vi "Read Interrupt.vi"(8 "error in (no error)":errorcluster, 11 "IO-4 Bricklet in":refnum<class "IO-4 Bricklet.lvclass">) -> (0 "error out":errorcluster, 2 "Interrupt":refnum<user-event>, 3 "IO-4 Bricklet out":refnum<class "IO-4 Bricklet.lvclass">)   [LabVIEW 2011, in "Tinkerforge.lvlib" / "IO-4 Bricklet.lvclass"]
uses:
  IO-4 Bricklet.lvclass
  Type Definitions/Interrupt.ctl
  IO-4 Bricklet.lvclass/IO-4 Bricklet.ctl
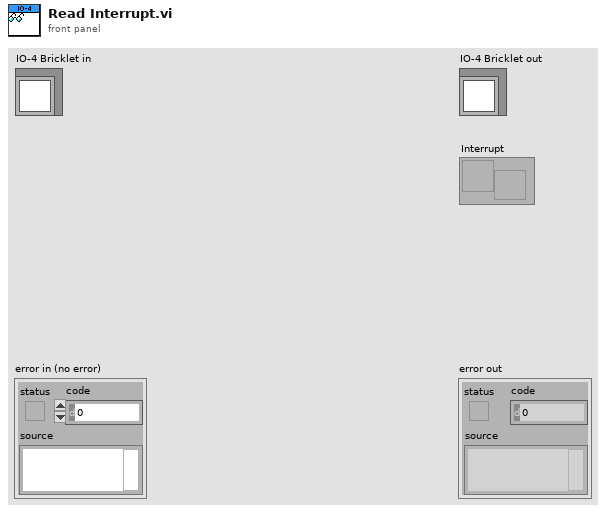
[diagram p1: front panel]
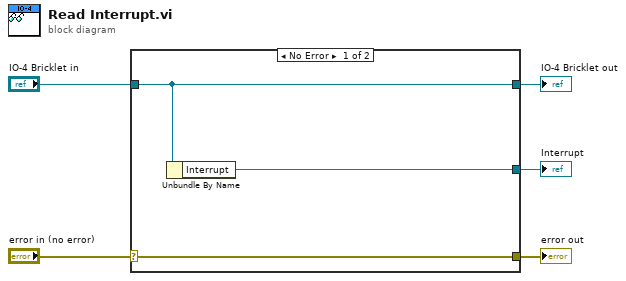
[diagram p0: block diagram]
diagram:
  n1 = case shown="No Error" "error in (no error)" {
    selector: "error in (no error)" -> [w8 w9]
    tunnel: [w8 w9] -> w4
    tunnel: [w7 w10] -> w2
    tunnel: "IO-4 Bricklet in" -> [w7 w10]
    tunnel: [w6 _] -> w1
    frame No Error {
      n2 = Unbundle By Name(w7) -> ("Interrupt"=w6:refnum<user-event>)
    }
    frame Error {
    }
  }
  "error out" <- w4
  "IO-4 Bricklet out" <- w2
  "Interrupt" <- w1
